vi "Helpdesk_Main.vi"() -> ()   [LabVIEW 2020]
uses:
  4c40cff2-8ddf-448c-9290-b0417c0ac7d6.vi
  Wolfram_class/Wolfram.lvclass
  C:/Projects/InterfacePresentation/Helpdesk/HelpInterface_interface/HelpInterface.lvclass
  Clippy_class/Clippy.lvclass
  C:/Projects/InterfacePresentation/PeriodicTrigger/PeriodicTrigger/Triggerable_interface/Triggerable.lvclass
  HelpInterface_interface/HelpInterface.lvclass
  PeriodicTrigger/PeriodicTrigger/PeriodicTrigger.lvlib
panel:
  in  "Help Desk Engine":enum16{"Wolfram Alpha", "Clippy"}(ring)
  out "Answer":string
  in  "Question":string
  in  "Help":bool
  out "Clippy":picture
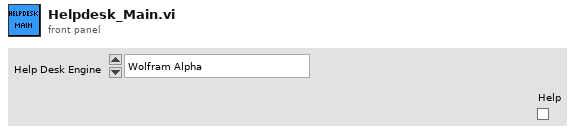
[diagram p1: front panel]
types:
  T1 = typedef "LVPoint32TypeDef.ctl" = cluster{"Horizontal":i32, "Vertical":i32}
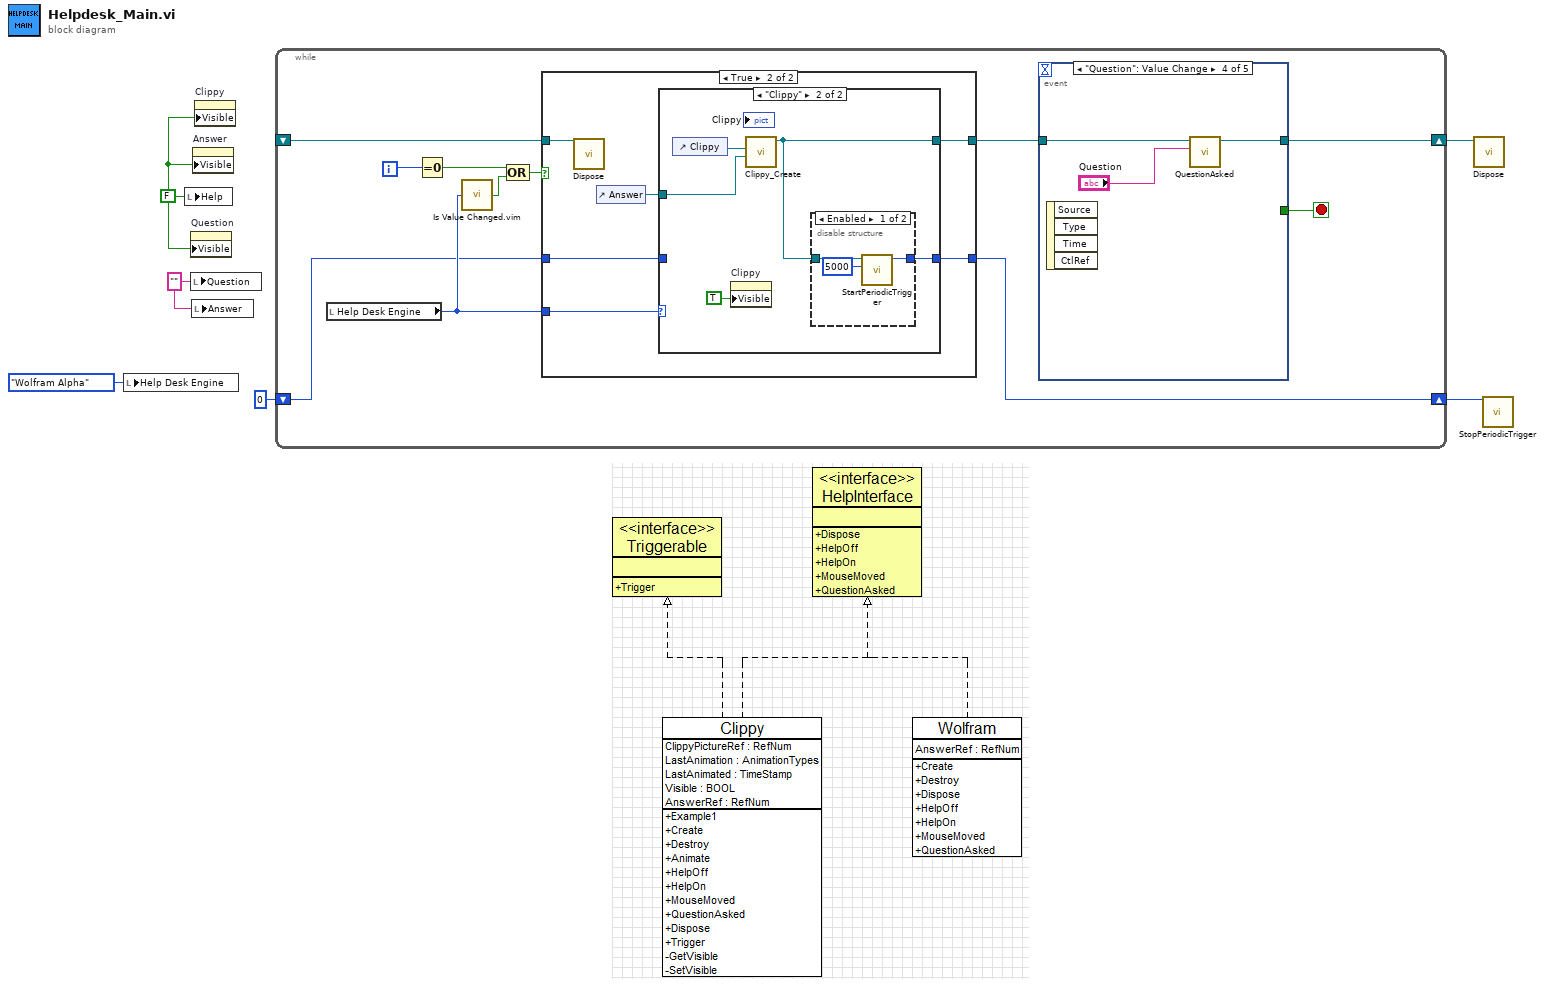
[diagram p0: block diagram]
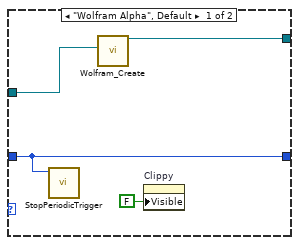
[diagram p3: hidden frame]
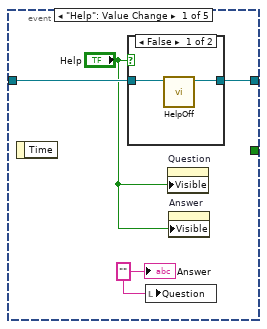
[diagram p5: hidden frame]
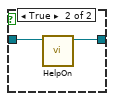
[diagram p6: hidden frame]
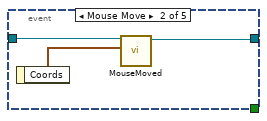
[diagram p7: hidden frame]
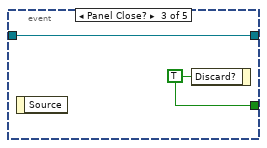
[diagram p8: hidden frame]
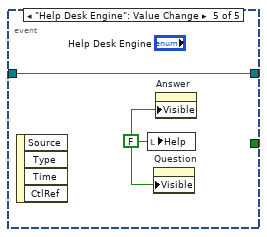
[diagram p9: hidden frame]
diagram:
  w4 = "" ("Question")
  w1 = FALSE ("Help")
  n1 = local write "Help Desk Engine"(enum16{"Wolfram Alpha", "Clippy"}."Wolfram Alpha" ("Help Desk Engine")) -> ()
  n2 = local write "Help"(w1) -> ()
  n3 = property on="Question" class="Str"("Visible"=w1) -> ()  [unwired: 2 in, 2 out]
  n4 = local write "Question"(w4) -> ()
  n5 = local write "Answer"(w4) -> ()
  n6 = property on="Answer" class="Str"("Visible"=w1) -> ()  [unwired: 2 in, 2 out]
  n7 = property on="Clippy" class="Pict"("Visible"=w1) -> ()  [unwired: 2 in, 2 out]
  n8 = while {
    shift-right: [w14] -> w5
    shift-left: _ -> [w13]
    shift-right: [w8] -> w3
    shift-left: u32 0 ("TriggerID") -> [w7]
    i -> [w12]
    stop <- w17 stop-if-true
    n9 = local read "Help Desk Engine"() -> (w15:enum16{"Wolfram Alpha", "Clippy"})
    n10 = Equal To 0?(x=w12) -> (x = 0?=w11:bool)
    n11 = call "Is Value Changed.vim"("value"=w15) -> ("changed or first call?"=w10:bool)
    n12 = Compound Arithmetic op=OR(w11, w10) -> (w9:bool)
    n13 = case shown="True" w9 {
      tunnel: [w19 w25] -> w16
      tunnel: w15 -> [_ w24]
      tunnel: w13 -> [w19 w23]
      tunnel: [w18 w21] -> w8
      tunnel: w7 -> [w18 w20]
      frame False {
      }
      frame True {
        n14 = call-dynamic "Dispose.vi"("object in"=w23) -> ()  [unwired: 9 in, 2 out]
        n15 = control-ref of="Answer"() -> (w22:refnum<vi>)
        n16 = case shown="\"Clippy\"" w24 {
          tunnel: [w29 w32] -> w25
          tunnel: w22 -> [w28 w33]
          tunnel: [w27 w31] -> w21
          tunnel: w20 -> [w27 _]
          frame "Wolfram Alpha", Default {
            n17 = call "StopPeriodicTrigger.vi"("TriggerID"=w27) -> ()  [unwired: 10 in, 1 out]
            n18 = call "Wolfram_Create.vi"("AnswerRef"=w28) -> ("reference out"=w29:refnum<class "Wolfram.lvclass">)  [unwired: 9 in, 1 out]
            n19 = property on="Clippy" class="Pict"("Visible"=FALSE) -> ()  [unwired: 2 in, 2 out]
          }
          frame "Clippy" {
            n20 = control-ref of="Clippy"() -> (w34:refnum<vi>)
            n21 = property on="Clippy" class="Pict"("Visible"=TRUE) -> ()  [unwired: 2 in, 2 out]
            n22 = call "Clippy_Create.vi"("AnswerRef"=w33, "ClippyPictureRef"=w34) -> ("reference out"=w32:refnum<class "Clippy.lvclass">)  [unwired: 8 in, 1 out]
            n23 = disable-structure shown="Enabled" {
              disable-tunnel: w32 -> [w37 _]
              disable-tunnel: [w35 _] -> w31
              frame Enabled {
                n24 = call "StartPeriodicTrigger.vi"("time (ms)"=5000, "Triggerable"=w37) -> ("TriggerID"=w35:u32)  [unwired: 8 in, 1 out]
              }
              frame Disabled {
              }
            }
          }
        }
      }
    }
    n25 = event shown="[3] \"Question\": Value Change" {
      selector: _ -> [_ _ _ _ _]
      dyn-events: _ -> [_ _ _ _ _]
      timeout: _ -> [_ _ _ _ _]
      tunnel: w16 -> [w41 w47 w49 w53 w54]
      tunnel: [_ _ w50 _ _] -> w17
      tunnel: [w40 w46 w49 w51 w54] -> w14
      event "Help": Value Change {
        w38 = "" ("Question")
        n26 = event-data() -> ()  [unwired: 1 in, 1 out]
        n27 = case shown="False" "Help" {
          tunnel: w41 -> [w43 w45]
          tunnel: [w42 w44] -> w40
          frame False {
            n28 = call-dynamic "HelpOff.vi"("object in"=w43) -> ("object out"=w42:refnum<class "HelpInterface.lvclass">)  [unwired: 9 in, 1 out]
          }
          frame True {
            n29 = call-dynamic "HelpOn.vi"("object in"=w45) -> ("object out"=w44:refnum<class "HelpInterface.lvclass">)  [unwired: 9 in, 1 out]
          }
        }
        n30 = local write "Question"(w38) -> ()
        n31 = property on="Question" class="Str"("Visible"="Help") -> ()  [unwired: 2 in, 2 out]
        n32 = property on="Answer" class="Str"("Visible"="Help") -> ()  [unwired: 2 in, 2 out]
        "Answer" <- w38
      }
      event Mouse Move {
        n33 = event-data() -> ("Coords"=w48:T1)  [unwired: 1 in]
        n34 = call-dynamic "MouseMoved.vi"("Point32"=w48, "object in"=w47) -> ("object out"=w46:refnum<class "HelpInterface.lvclass">)  [unwired: 8 in, 1 out]
      }
      event Panel Close? {
        w50 = TRUE ("Discard?")
        n35 = event-data() -> ()  [unwired: 1 in, 1 out]
        n36 = event-data("Discard?"=w50) -> ()  [unwired: 1 in, 1 out]
      }
      event "Question": Value Change {
        n37 = event-data() -> ()  [unwired: 1 in, 4 out]
        n38 = call-dynamic "QuestionAsked.vi"("Question"="Question", "object in"=w53) -> ("object out"=w51:refnum<class "HelpInterface.lvclass">)  [unwired: 8 in, 1 out]
      }
      event "Help Desk Engine": Value Change {
        w55 = FALSE ("Help")
        n39 = event-data() -> ()  [unwired: 1 in, 4 out]
        n40 = local write "Help"(w55) -> ()
        n41 = property on="Question" class="Str"("Visible"=w55) -> ()  [unwired: 2 in, 2 out]
        n42 = property on="Answer" class="Str"("Visible"=w55) -> ()  [unwired: 2 in, 2 out]
      }
    }
  }
  n43 = call-dynamic "Dispose.vi"("object in"=w5) -> ()  [unwired: 9 in, 2 out]
  n44 = call "StopPeriodicTrigger.vi"("TriggerID"=w3) -> ()  [unwired: 10 in, 1 out]
